vi "writeToXML.vi"(8 "error in (no error)":errorcluster, 10 "ClassLabel":string, 11 "MccDebug in":refnum<class "MccDebug.lvclass">) -> (0 "error out":errorcluster, 2 "XML out":string, 3 "MccDebug out":refnum<class "MccDebug.lvclass">)   [LabVIEW 2022 SP3, in "TCSDataDefinitions.lvlib" / "TCSMountControlCommand.lvlib" / "CommandsForAllAxes.lvlib" / "MccDebug.lvclass"]
uses:
  MccDebug.lvclass
  MccDebug.lvclass/MccDebug.ctl
  CommandsForAllAxes.lvclass
  <userlib>/Common/XML/XMLGenerator/XMLGenerator.lvclass
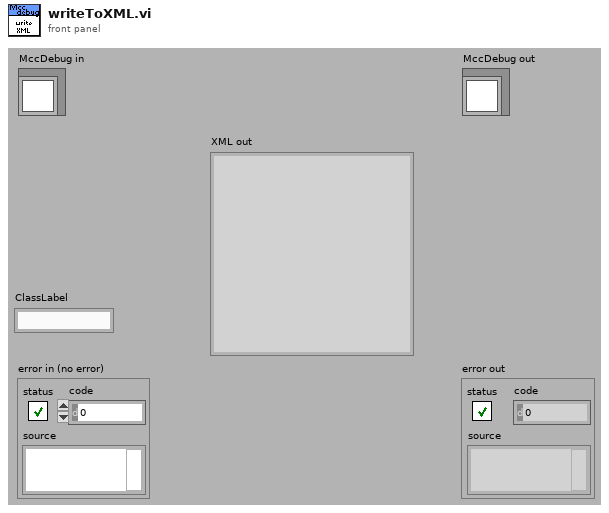
[diagram p1: front panel]
types:
  T1 = typedef "TCSDataDefinitions.lvlib/TCSCommand.lvlib/TCSDebuLevelTypes.ctl" = enum16{"0", "1", "2", "3", "4", "5", "6", "7", "8", "9", "10"}
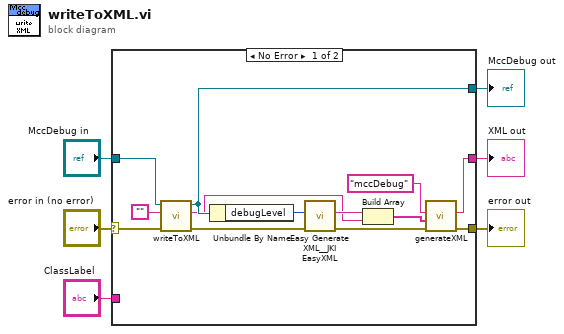
[diagram p0: block diagram]
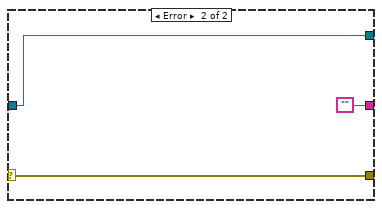
[diagram p2: hidden frame]
diagram:
  n1 = case shown="No Error" "error in (no error)" {
    selector: "error in (no error)" -> [w9 w22]
    tunnel: [w8 w22] -> w5
    tunnel: [w17 w21] -> w3
    tunnel: "MccDebug in" -> [w19 w21]
    tunnel: "ClassLabel" -> [_ _]
    tunnel: [w7 ""] -> w1
    frame No Error {
      n2 = call-parent "writeToXML.vi"("error in (no error)"=w9, "ClassLabel"="", "CommandsForAllAxes in"=w19) -> ("error out"=w15:errorcluster, "XMLout"=w13:string, "CommandsForAllAxes out"=w17:refnum<class "MccDebug.lvclass">)  [unwired: 6 in]
      n3 = Unbundle By Name(w17) -> ("debugLevel"=w16:T1)
      n4 = call <vilib>:"Easy Generate XML__JKI EasyXML.vi"("error in (no error)"=w15, "LabVIEW Data"=w16) -> ("error out"=w10:errorcluster, "XML String"=w14:string)  [unwired: 8 in]
      n5 = Build Array(w14, w13) -> (w12:string[])
      n6 = call <userlib>:"generateXML.vi"("error in"=w10, "childrenXML"=w12, "elementName"="mccDebug" ("Class Label")) -> ("error out"=w8:errorcluster, "XML out"=w7:string)  [unwired: 6 in, 1 out]
    }
    frame Error {
    }
  }
  "error out" <- w5
  "MccDebug out" <- w3
  "XML out" <- w1
